vi "Constellation graph.vi"() -> ()   [LabVIEW 2026]
panel:
  out "Constellation graph":cluster{"Y":dbl[], "Y":dbl[]}[](graph)
  in  "Odd bits":dbl[](array[numeric])
  in  "Even bits":dbl[](array[numeric])
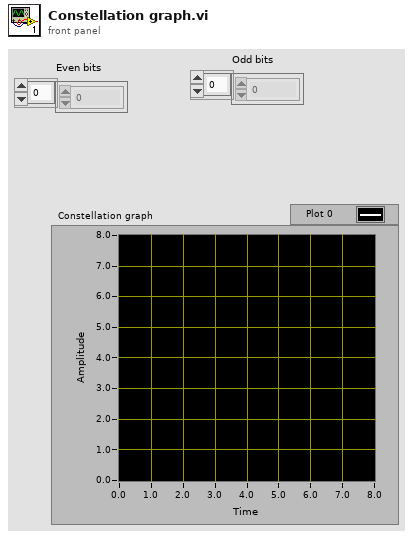
[diagram p1: front panel]
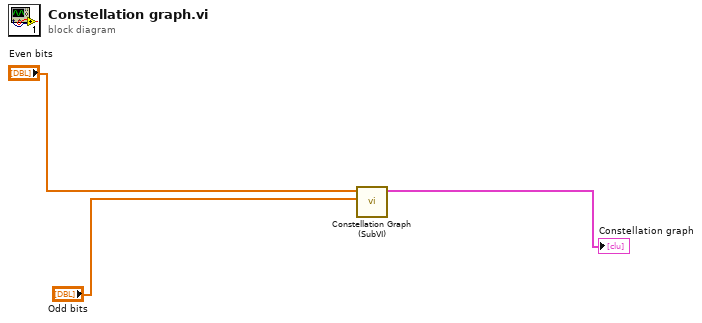
[diagram p0: block diagram]
diagram:
  n1 = call "Constellation Graph (SubVI).vi"("Odd bits"="Odd bits", "Even bits"="Even bits") -> ("Constellation graph"=→"Constellation graph":cluster{"Y":dbl[], "Y":dbl[]}[])  [unwired: 9 in]
